vi "TCP-Measure RTT.vi"(0 "Name":string, 2 "Parent VI":refnum<vi>, 7 "Address in":string, 11 "string ack":bool) -> (8 "result":string)   [LabVIEW 2020]
uses:
  <extravilib>/ChannelInstances/Stream-dbl/Read With Abort.vi
  TCP Write.vi
  <extravilib>/ChannelInstances/Stream-dbl/Write With Abort.vi
  <extravilib>/ChannelInstances/Stream-dbl/EndpointRead.vi
  <extravilib>/ChannelInstances/Stream-dbl/Endpoint.vi
  <extravilib>/ChannelInstances/Stream-dbl/Instantiate.vi
  <extravilib>/ChannelInstances/Stream-dbl/)Channel.vi
  <resource>/ChannelSupport/_ChannelSupport/WaitIfNeeded.vi
  TCP-Check Result.vi
  <extravilib>/ChannelInstances/Stream-dbl.lvlib
  <vilib>/Analysis/NI_AALBase.lvlib
panel:
  in  "test which":enum32{"UDP", "TCP"}(radio)=enum."TCP"
  out "TCP":string
  out "timing":T1(graph)
  out "Max (us)":dbl
  out "Min (us)":dbl
  out "Std. Dev. (us)":dbl
  out "Mean (us)":dbl
  in  "Finished Button":bool
  in  "Start Button":bool
  in  "Number to send":i32=10000
  out "Sent":i32
  out "UDP":string
  out "finished":errorcluster
  in  "Stop Button":bool
  # "TCP Utilities"
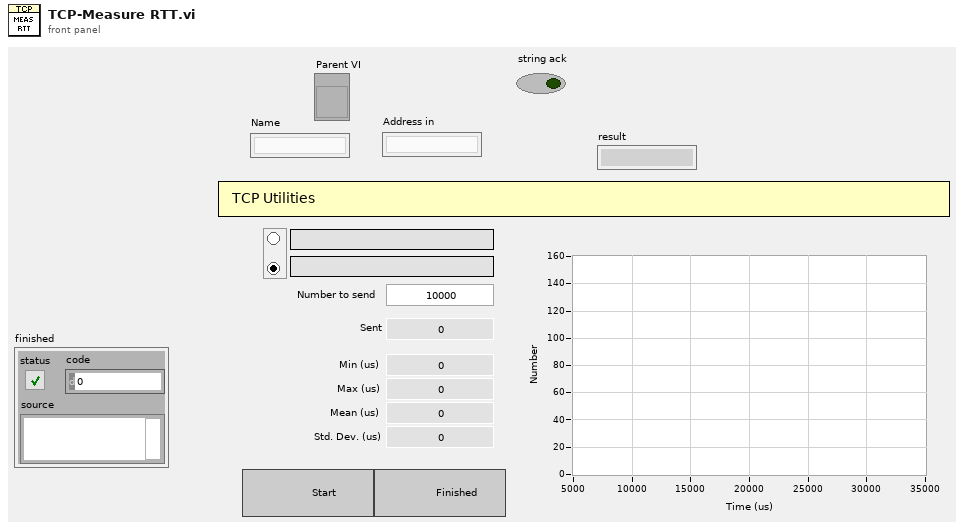
[diagram p1: front panel]
types:
  T1 = cluster{"X Values":dbl[], "Histogram: h(x)":i32[]}
  T2 = typedef "Stream-dbl.lvlib/)Channel.ctl" = refnum<queue>
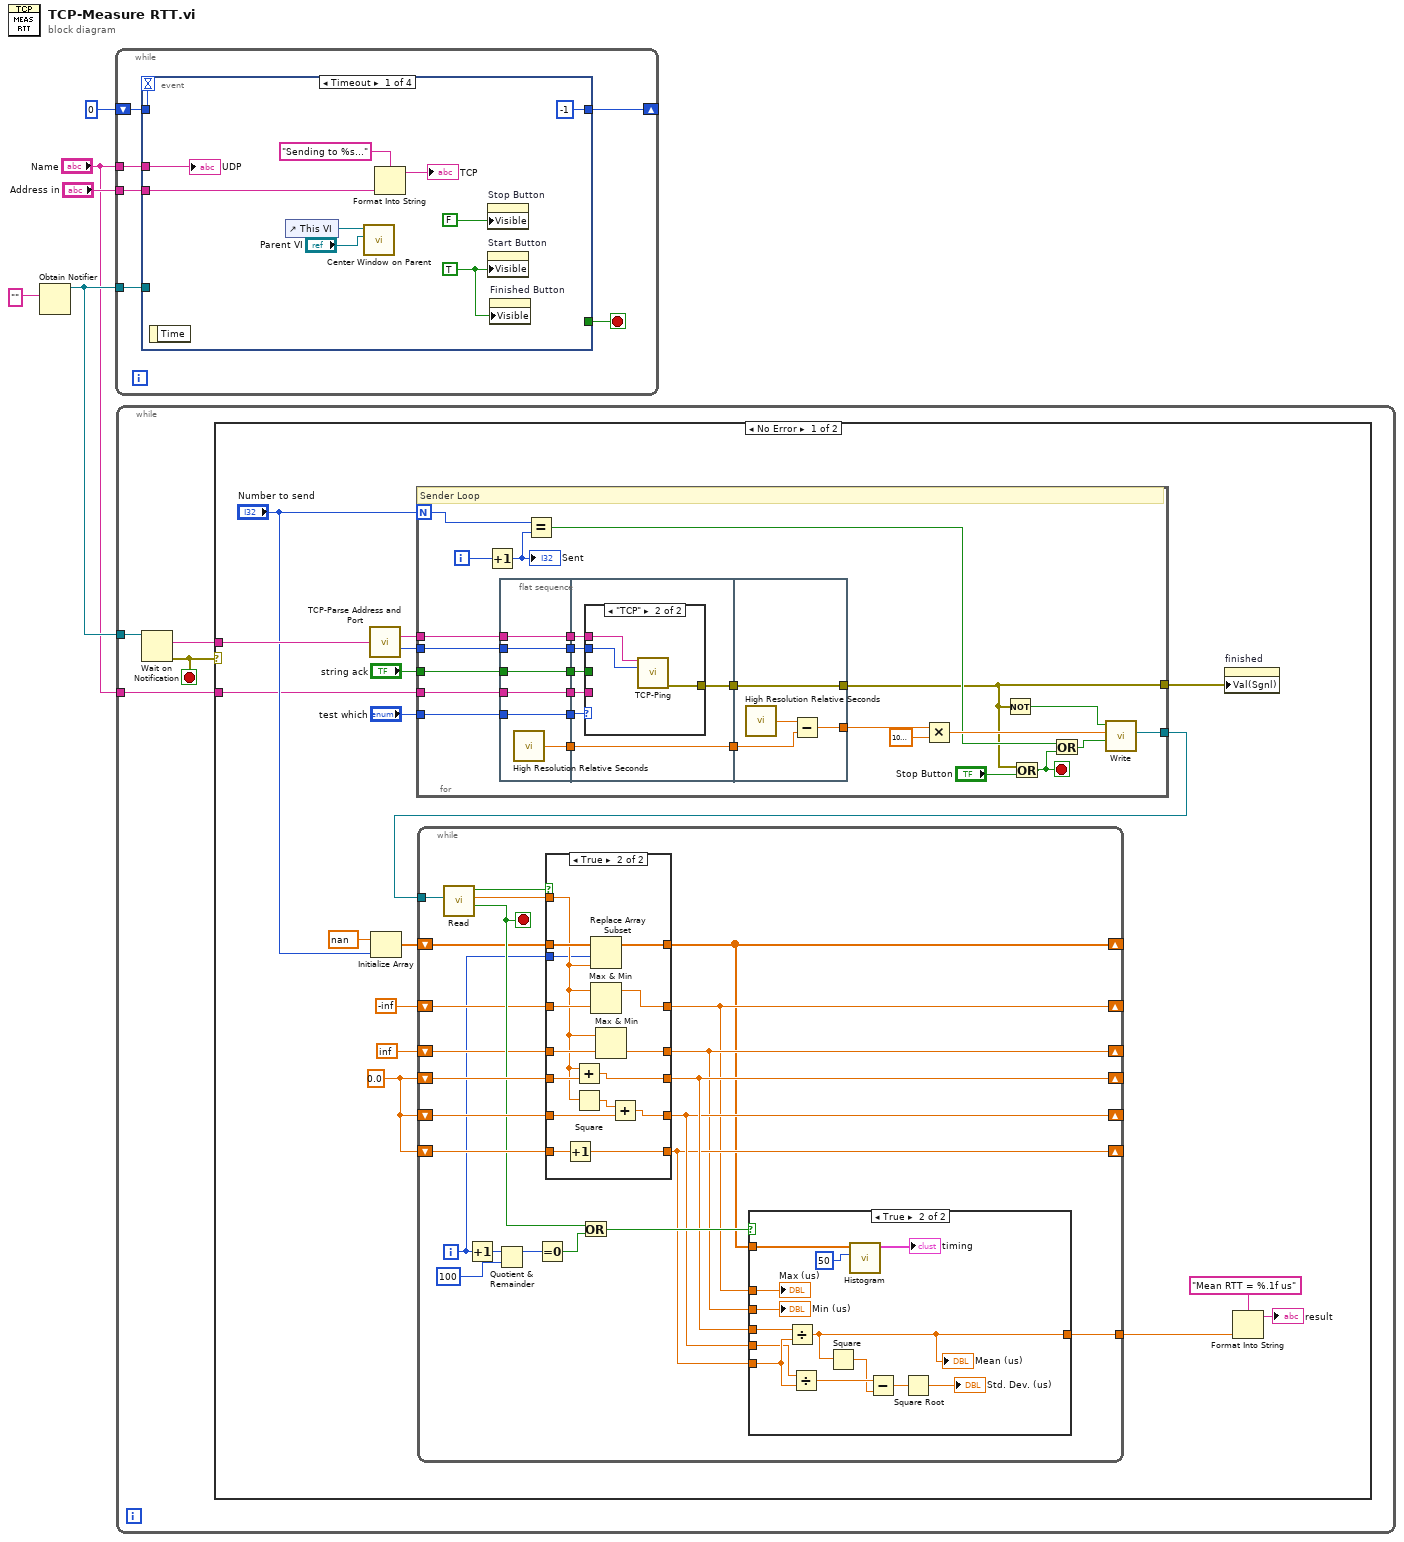
[diagram p0: block diagram]
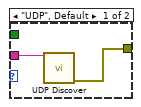
[diagram p2: hidden frame]
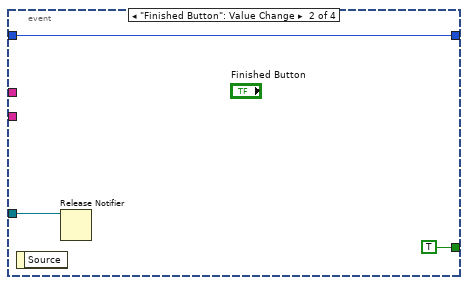
[diagram p6: hidden frame]
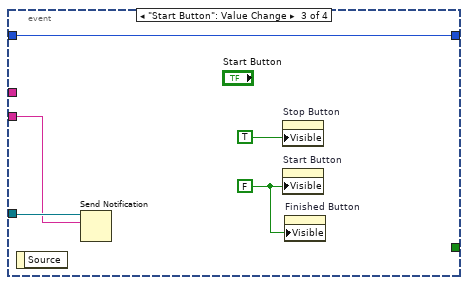
[diagram p7: hidden frame]
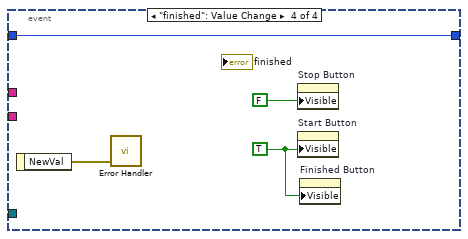
[diagram p8: hidden frame]
diagram:
  n1 = Obtain Notifier(notification data type="") -> (notifier out=w3:refnum<notifier>)  [unwired: 3 in, 2 out]
  n2 = while {
    shift-right: [w10] -> _
    shift-left: 0 -> [w11]
    tunnel: w3 -> [w8]
    tunnel: "Address in" -> [w7]
    tunnel: "Name" -> [w6]
    stop <- w9 stop-if-true
    n3 = event shown="[0] Timeout" {
      selector: _ -> [_ _ _ _]
      dyn-events: _ -> [_ _ _ _]
      timeout: w11 -> [_ _ _ _]
      tunnel: w11 -> [_ w23 w28 w32]
      tunnel: [-1 w23 w28 w32] -> w10
      tunnel: [_ TRUE _ _] -> w9
      tunnel: w8 -> [_ w21 w27 _]
      tunnel: w7 -> [w16 _ w26 _]
      tunnel: w6 -> [w12 _ _ _]
      event Timeout {
        w14 = TRUE
        n4 = event-data() -> ()  [unwired: 1 in, 1 out]
        n5 = control-ref of="This VI"() -> (w19:refnum<vi>)
        n6 = call "Center Window on Parent.vi"("Parent VI"="Parent VI", "VI in"=w19) -> ()  [unwired: 8 in, 2 out]
        n7 = Format Into String(format string="Sending to %s...", w16) -> (resulting string=→"TCP":string)  [unwired: 2 in, 1 out]
        n8 = property on="Stop Button" class="Bool"("Visible"=FALSE) -> ()  [unwired: 2 in, 2 out]
        n9 = property on="Start Button" class="Bool"("Visible"=w14) -> ()  [unwired: 2 in, 2 out]
        n10 = property on="Finished Button" class="Bool"("Visible"=w14) -> ()  [unwired: 2 in, 2 out]
        "UDP" <- w12
      }
      event "Finished Button": Value Change {
        n11 = event-data() -> ()  [unwired: 1 in, 1 out]
        n12 = Release Notifier(notifier=w21) -> ()  [unwired: 2 in, 3 out]
      }
      event "Start Button": Value Change {
        w24 = FALSE
        n13 = event-data() -> ()  [unwired: 1 in, 1 out]
        n14 = Send Notification(notification=w26, notifier=w27) -> ()  [unwired: 1 in, 2 out]
        n15 = property on="Stop Button" class="Bool"("Visible"=TRUE) -> ()  [unwired: 2 in, 2 out]
        n16 = property on="Start Button" class="Bool"("Visible"=w24) -> ()  [unwired: 2 in, 2 out]
        n17 = property on="Finished Button" class="Bool"("Visible"=w24) -> ()  [unwired: 2 in, 2 out]
      }
      event "finished": Value Change {
        w29 = TRUE
        n18 = event-data() -> ("NewVal"=w31:errorcluster)  [unwired: 1 in]
        n19 = call "Error Handler.vi"("error in (no error)"=w31) -> ()  [unwired: 12 in, 3 out]
        n20 = property on="Stop Button" class="Bool"("Visible"=FALSE) -> ()  [unwired: 2 in, 2 out]
        n21 = property on="Start Button" class="Bool"("Visible"=w29) -> ()  [unwired: 2 in, 2 out]
        n22 = property on="Finished Button" class="Bool"("Visible"=w29) -> ()  [unwired: 2 in, 2 out]
      }
    }
  }
  n23 = while {
    tunnel: w3 -> [w36]
    tunnel: "Name" -> [w33]
    stop <- w35 stop-if-true
    n24 = Wait on Notification(notifier=w36) -> (notification=w34:string, error out=w35:errorcluster)  [unwired: 3 in, 2 out]
    n25 = case shown="No Error" w35 {
      tunnel: w34 -> [w53 _]
      tunnel: w33 -> [w38 _]
      frame No Error {
        w51 = 0.0
        n26 = call "TCP-Parse Address and Port.vi"("Address in"=w53) -> ("Address"=w47:string, "Port"=w48:i32)  [unwired: 12 in, 1 out]
        n27 = Initialize Array(nan, "Number to send") -> (w40:dbl[])
        n28 = for {
          N: "Number to send" -> [w67]
          tunnel: w47 -> [w78]
          tunnel: [w72] -> w52
          tunnel: w48 -> [w62]
          tunnel: [w60] -> w46
          tunnel: "test which" -> [w58]
          tunnel: w38 -> [w56]
          tunnel: "string ack" -> [w54]
          i -> [w77]
          stop <- w66 stop-if-true
          # "Sender Loop"
          n29 = Increment(x=w77) -> (x+1=w68:i32)
          "Sent" <- w68
          n30 = flat-sequence {
            tunnel: w78 -> [w85]
            tunnel: [w85] -> w76
            tunnel: [w84] -> w75
            tunnel: [w83] -> w63
            tunnel: w62 -> [w83]
            tunnel: [w82] -> w59
            tunnel: w58 -> [w82]
            tunnel: [w81] -> w57
            tunnel: w56 -> [w81]
            tunnel: [w80] -> w55
            tunnel: w54 -> [w80]
            tunnel: w76 -> [w91]
            tunnel: w75 -> [w92]
            tunnel: [w92] -> w74
            tunnel: w63 -> [w90]
            tunnel: [w89] -> w61
            tunnel: w59 -> [w88]
            tunnel: w57 -> [w87]
            tunnel: w55 -> [w86]
            tunnel: w74 -> [w100]
            tunnel: [w99] -> w73
            tunnel: [w98] -> w60
            tunnel: w61 -> [w98]
            frame #0 {
              n31 = call <vilib>:"High Resolution Relative Seconds.vi"() -> ("relative seconds"=w84:dbl)
            }
            frame #1 {
              n32 = case shown="\"TCP\"" w88 {
                tunnel: w91 -> [_ w97]
                tunnel: w90 -> [_ w96]
                tunnel: [w93 w95] -> w89
                tunnel: w87 -> [w94 _]
                tunnel: w86 -> [_ _]
                frame "UDP", Default {
                  n33 = call "UDP Discover.vi"("Name"=w94) -> ("error out"=w93:errorcluster)  [unwired: 10 in, 4 out]
                }
                frame "TCP" {
                  n34 = call "TCP-Ping.vi"("IP Address"=w97, "Port"=w96) -> ("error out"=w95:errorcluster)  [unwired: 13 in]
                }
              }
            }
            frame #2 {
              n35 = call <vilib>:"High Resolution Relative Seconds.vi"() -> ("relative seconds"=w101:dbl)
              n36 = Subtract(x=w101, y=w100) -> (x-y=w99:dbl)
            }
          }
          n37 = Equal?(x=w67, y=w68) -> (x = y?=w65:bool)
          n38 = Multiply(x=w73, y=1000000.0) -> (x*y=w70:dbl)
          n39 = Not(x=w60) -> (.not. x?=w71:bool)
          n40 = Or(x=w60, y="Stop Button") -> (x .or. y?=w66:bool)
          n41 = Or(x=w65, y=w66) -> (x .or. y?=w64:bool)
          n42 = call <extravilib>:"Write.vi"("last element? (F)"=w64, "element"=w70, "element valid? (T)"=w71) -> ("channel"=w72:T2)  [unwired: 6 in, 2 out]
        }
        n43 = while {
          tunnel: w52 -> [w124]
          shift-right: [w112] -> _
          shift-left: w51 -> [w121]
          shift-right: [w111] -> _
          shift-left: w51 -> [w120]
          shift-right: [w110] -> _
          shift-left: w51 -> [w119]
          shift-right: [w106] -> _
          shift-left: -inf -> [w109]
          shift-right: [w107] -> _
          shift-left: inf -> [w108]
          tunnel: [w105] -> w45
          shift-right: [w102] -> _
          shift-left: w40 -> [w104]
          i -> [w103]
          stop <- w114 stop-if-true
          n44 = call <extravilib>:"Read.vi"("channel"=w124) -> ("last element?"=w114:bool, "element"=w122:dbl, "element valid?"=w123:bool)  [unwired: 6 in, 2 out]
          n45 = Increment(x=w103) -> (x+1=w116:i32)
          n46 = Quotient & Remainder(x=w116, y=100) -> (x-y*floor(x/y)=w117:i32)  [unwired: 1 out]
          n47 = Equal To 0?(x=w117) -> (x = 0?=w115:bool)
          n48 = case shown="True" w123 {
            tunnel: w122 -> [_ w146]
            tunnel: w121 -> [w143 w158]
            tunnel: w120 -> [w142 w154]
            tunnel: w119 -> [w141 w156]
            tunnel: [w143 w157] -> w112
            tunnel: [w142 w152] -> w111
            tunnel: [w141 w155] -> w110
            tunnel: w109 -> [w140 w151]
            tunnel: [w140 w150] -> w106
            tunnel: w108 -> [w139 w149]
            tunnel: [w139 w148] -> w107
            tunnel: w104 -> [w138 w147]
            tunnel: w103 -> [_ w145]
            tunnel: [w138 w144] -> w102
            frame False {
            }
            frame True {
              n49 = Increment(x=w156) -> (x+1=w155:dbl)
              n50 = Add(x=w146, y=w158) -> (x+y=w157:dbl)
              n51 = Square(x=w146) -> (x^2=w153:dbl)
              n52 = Replace Array Subset(array=w147, new element=w146, index=w145) -> (w144:dbl[])
              n53 = Max & Min(x=w146, y=w151) -> (max(x,y)=w150:dbl)  [unwired: 1 out]
              n54 = Max & Min(x=w146, y=w149) -> (min(x,y)=w148:dbl)  [unwired: 1 out]
              n55 = Add(x=w153, y=w154) -> (x+y=w152:dbl)
            }
          }
          n56 = Or(x=w114, y=w115) -> (x .or. y?=w113:bool)
          n57 = case shown="True" w113 {
            tunnel: w112 -> [_ w137]
            tunnel: w111 -> [_ w135]
            tunnel: w110 -> [_ w136]
            tunnel: w107 -> [_ w129]
            tunnel: w106 -> [_ w130]
            tunnel: [_ w128] -> w105
            tunnel: w102 -> [_ w125]
            frame False {
            }
            frame True {
              n58 = Divide(x=w137, y=w136) -> (x/y=w128:dbl)
              "Mean (us)" <- w128
              n59 = Divide(x=w135, y=w136) -> (x/y=w134:dbl)
              n60 = Square(x=w128) -> (x^2=w133:dbl)
              n61 = call <vilib>:"Histogram.vi"("intervals"=50, "X"=w125) -> ("Histogram Graph"=→"timing":T1)  [unwired: 6 in, 3 out]
              n62 = Subtract(x=w134, y=w133) -> (x-y=w132:dbl)
              n63 = Square Root(x=w132) -> (sqrt(x)=→"Std. Dev. (us)":dbl)
              "Max (us)" <- w130
              "Min (us)" <- w129
            }
          }
        }
        n64 = property on="finished" class="Clust (strict)"("Val(Sgnl)"=w46) -> ()  [unwired: 2 in, 2 out]
        n65 = Format Into String(format string="Mean RTT = %.1f us", w45) -> (resulting string=→"result":string)  [unwired: 2 in, 1 out]
      }
      frame Error {
      }
    }
  }
